vi "FPWindow.vi"(8 "error in":errorcluster, 11 "VI Refnum":refnum<vi>) -> (0 "error out":errorcluster, 3 "FPWindow out":refnum<class "FPWindow.lvclass">)   [LabVIEW 2014, in "Raspberry Pi Compatible Compiler for LabVIEW.lvlib" / "FPWindow.lvclass"]
uses:
  FPWindow.lvclass
  FPWindow.lvclass/FPWindow.ctl
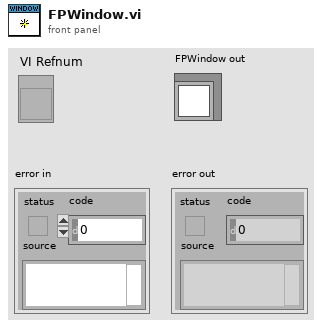
[diagram p1: front panel]
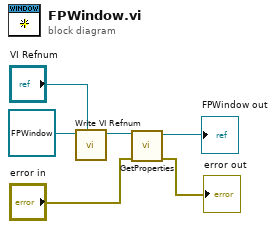
[diagram p0: block diagram]
diagram:
  n1 = call "Write VI Refnum.vi"("VI Refnum"="VI Refnum", "FPWindow in"=refnum<class "FPWindow.lvclass"> refnum) -> ("FPWindow out"=w4:refnum<class "FPWindow.lvclass">)  [unwired: 7 in]
  n2 = call "GetProperties.vi"("error in"="error in", "FPWindow in"=w4) -> ("error out"=→"error out":errorcluster, "FPWindow out"=→"FPWindow out":refnum<class "FPWindow.lvclass">)  [unwired: 8 in]
